vi "Enable with Default Values.vi"(8 "error in (no error)":errorcluster, 11 "LPS Barometer in":refnum<class "LPS Barometric Pressure Sensor.lvclass">) -> (0 "error out":errorcluster, 3 "LPS Barometer out":refnum<class "LPS Barometric Pressure Sensor.lvclass">)   [LabVIEW 2020, in "LPS Barometric Pressure Sensor.lvclass"]
doc: "Enables continuous acquisition with a 12.5Hz data rate."
uses:
  LPS Barometric Pressure Sensor.lvclass
  LINX I2C/LINX I2C.lvclass
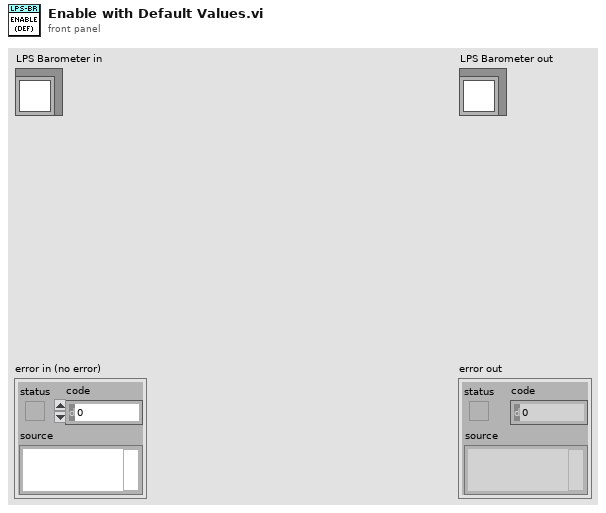
[diagram p1: front panel]
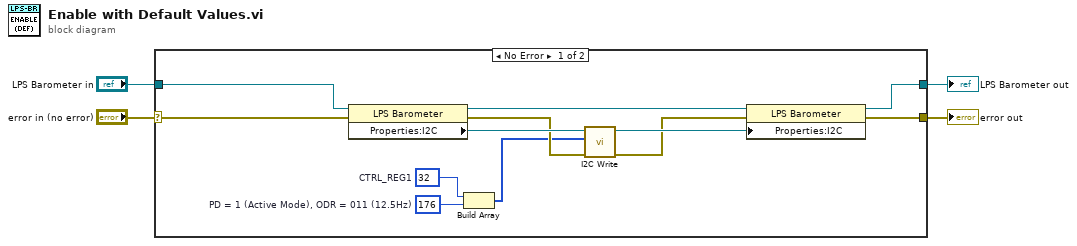
[diagram p0: block diagram]
diagram:
  n1 = case shown="No Error" "error in (no error)" {
    selector: "error in (no error)" -> [w9 w18]
    tunnel: [w8 w18] -> w3
    tunnel: [w14 w17] -> w1
    tunnel: "LPS Barometer in" -> [w16 w17]
    frame No Error {
      w6 = u8 176  # PD = 1 (Active Mode), ODR = 011 (12.5Hz)
      w7 = u8 32  # CTRL_REG1
      n2 = property class="LPS Barometer"(reference=w16, error in=w9) -> (reference out=w15:refnum<class "LPS Barometric Pressure Sensor.lvclass">, error out=w11:errorcluster, "Properties:I2C"=w13:refnum<class "LINX I2C.lvclass">)
      n3 = Build Array(w7, w6) -> (w5:u8[])
      n4 = call "I2C Write.vi"("error in (no error)"=w11, "Bytes to Write"=w5, "LINX I2C in"=w13) -> ("error out"=w10:errorcluster, "LINX I2C out"=w12:refnum<class "LINX I2C.lvclass">)  [unwired: 7 in]
      n5 = property class="LPS Barometer"(reference=w15, error in=w10, "Properties:I2C"=w12) -> (reference out=w14:refnum<class "LPS Barometric Pressure Sensor.lvclass">, error out=w8:errorcluster)
    }
    frame Error {
    }
  }
  "error out" <- w3
  "LPS Barometer out" <- w1
